vi "Get ColumnName Alais Name.vi"(8 "error in (no error)":errorcluster, 10 "TableName":string="Results", 11 "SQLite in":refnum<class "SQLite.lvclass">) -> (0 "error out":errorcluster, 2 "Columnname_Alais":string[](array[string]), 3 "SQLite out":refnum<class "SQLite.lvclass">)   [LabVIEW 2017, in "SQLite.lvclass"]
uses:
  SQLite.lvclass
  \\vmware-host\Shared Folders/D/Dev/NJAL/OP140/OP140_NJAL_valve_EOL_Test_20210806/Source_Public/DataBase/Top DB/TopDBClass.lvclass
  <userlib>/LabSQL/LabSQL.lvlib
  <userlib>/sushu/sushu.lvlib
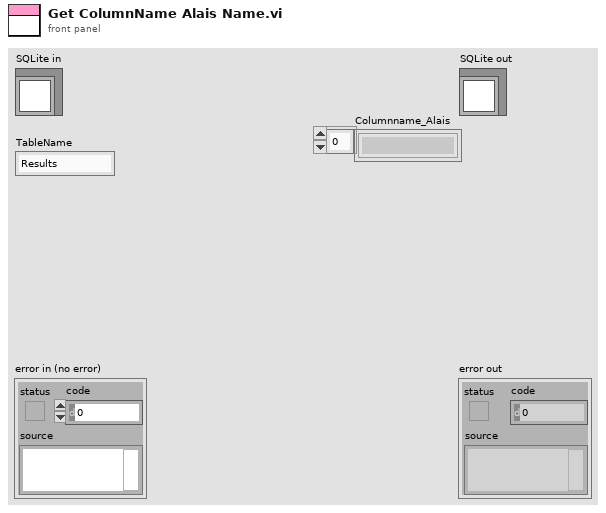
[diagram p1: front panel]
types:
  T1 = enum16{"Other", "SQL2008", "SQLite", "Access", "MySQL"}
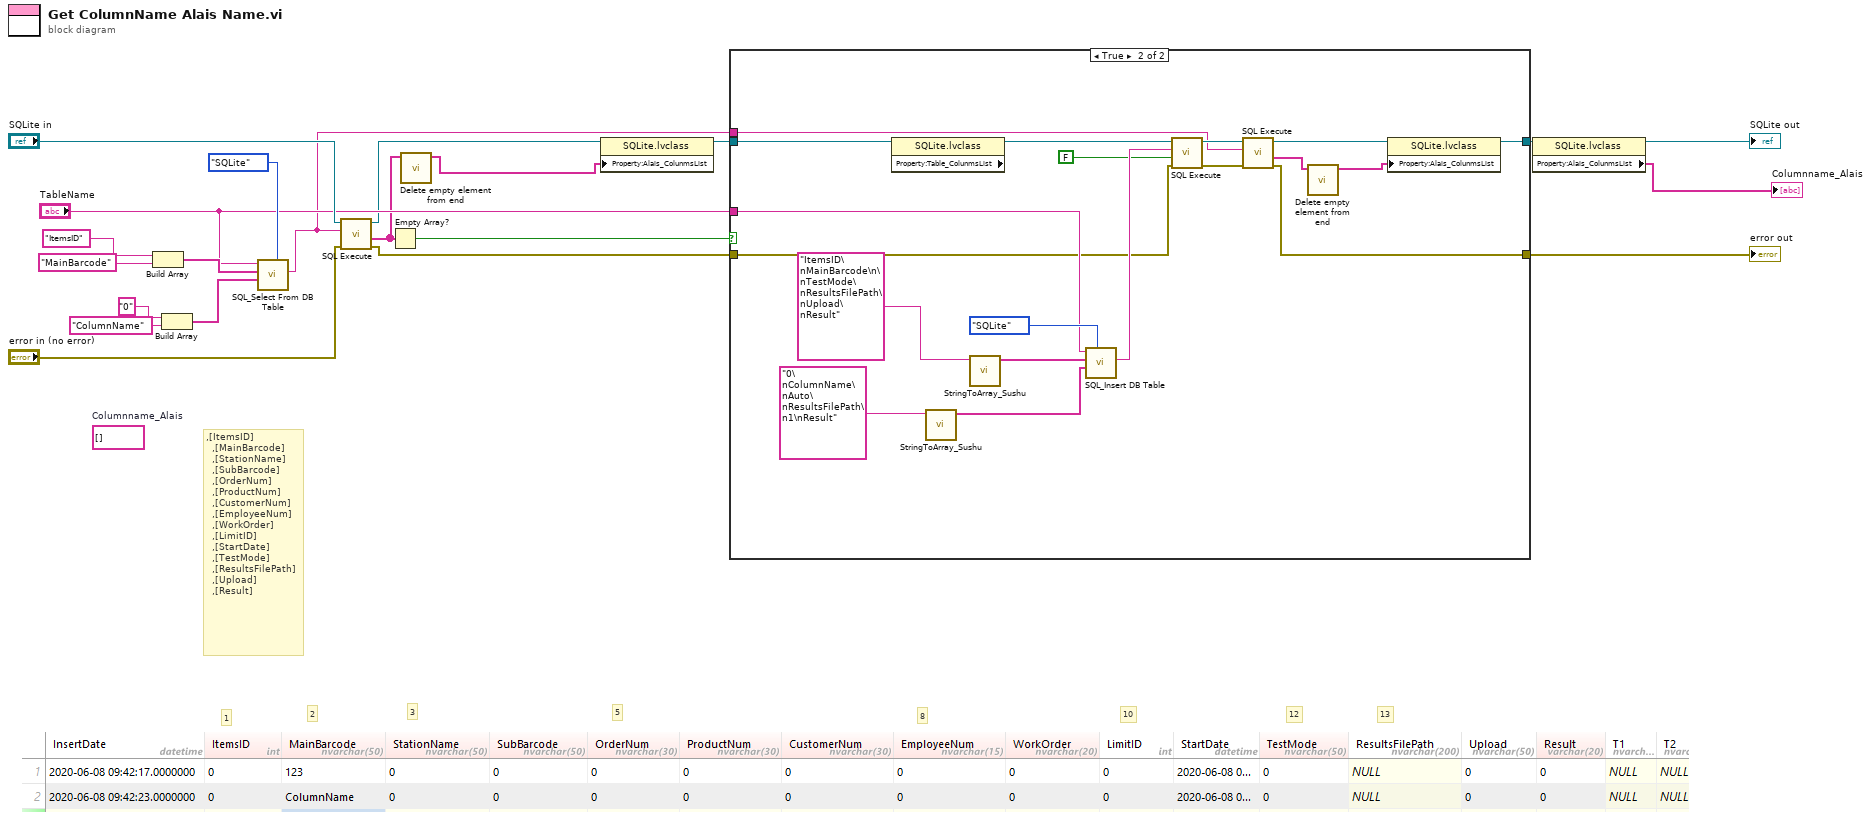
[diagram p0: block diagram]
diagram:
  (unwired) string[] []  # Columnname_Alais
  # "13"
  # "12"
  # "10"
  # "8"
  # "5"
  # "3"
  # "2"
  # "1"
  # ",[ItemsID]\n\t\t,[MainBarcode]\n\t\t,[StationName]\n\t\t,[SubBarcode]\n\t\t,[OrderNum]\n\t\t,[ProductNum]\n\t\t,[CustomerNum]\n\t\t,[EmployeeNum]\n\t\t,[WorkOrder]\n\t\t,[LimitID]\n\t\t,[StartDate]\n\t\t,[TestMode]\n\t\t,[ResultsFilePath]\n\t\t,[Upload]\n\t\t,[Result]"
  n1 = Build Array("ItemsID" ("element"), "MainBarcode" ("element")) -> (w18:string[])
  n2 = Build Array("0" ("element"), "ColumnName" ("element")) -> (w19:string[])
  n3 = call <userlib>:"SQL_Select From DB Table.vi"("DB Type"=T1."SQLite", "ColumnsValue"=w19, "ColumnsNameList"=w18, "TableName"="TableName") -> ("Select SQL CMD"=w8:string)  [unwired: 7 in]
  n4 = call-dynamic "SQL Execute.vi"("error in (no error)"="error in (no error)", "Command Text"=w8, "HostDB in"="SQLite in") -> ("error out"=w11:errorcluster, "FirstRow"=w6:string[], "HostDB out"=w3:refnum<class "SQLite.lvclass">)  [unwired: 4 in, 2 out]
  n5 = Empty Array?(array=w6) -> (empty?=w12:bool)
  n6 = call "Delete empty element from end.vi"("Columnname_Alais"=w6) -> ("reversed array"=w4:string[])  [unwired: 10 in]
  n7 = property class="SQLite.lvclass"(reference=w3, "Property:Alais_ColunmsList"=w4) -> (reference out=w5:refnum<class "SQLite.lvclass">)  [unwired: 1 in, 1 out]
  n8 = case shown="True" w12 {
    tunnel: w5 -> [w23 w39]
    tunnel: [w23 w25] -> w7
    tunnel: w11 -> [w22 w32]
    tunnel: [w22 w28] -> w10
    tunnel: "TableName" -> [_ w37]
    tunnel: w8 -> [_ w30]
    frame False {
    }
    frame True {
      n9 = property class="SQLite.lvclass" props=["Property:Table_ColunmsList"](reference=w39) -> (reference out=w38:refnum<class "SQLite.lvclass">)  [unwired: 1 in, 2 out]
      n10 = call <userlib>:"StringToArray_Sushu.vi"("State Queue"="0\nColumnName\nAuto\nResultsFilePath\n1\nResult") -> ("Array"=w33:string[])  [unwired: 8 in, 2 out]
      n11 = call <userlib>:"StringToArray_Sushu.vi"("State Queue"="ItemsID\nMainBarcode\n\nTestMode\nResultsFilePath\nUpload\nResult") -> ("Array"=w36:string[])  [unwired: 8 in, 2 out]
      n12 = call <userlib>:"SQL_Insert DB Table.vi"("DB Type"=T1."SQLite", "ColumnsValue"=w33, "ColumnsName"=w36, "Table Name"=w37) -> ("Insert DB String"=w42:string)  [unwired: 7 in]
      n13 = call-dynamic "SQL Execute.vi"("error in (no error)"=w32, "Return Data (T)"=FALSE, "Command Text"=w42, "HostDB in"=w38) -> ("error out"=w29:errorcluster, "HostDB out"=w31:refnum<class "SQLite.lvclass">)  [unwired: 3 in, 3 out]
      n14 = call-dynamic "SQL Execute.vi"("error in (no error)"=w29, "Command Text"=w30, "HostDB in"=w31) -> ("error out"=w28:errorcluster, "FirstRow"=w27:string[], "HostDB out"=w26:refnum<class "SQLite.lvclass">)  [unwired: 4 in, 2 out]
      n15 = call "Delete empty element from end.vi"("Columnname_Alais"=w27) -> ("reversed array"=w24:string[])  [unwired: 10 in]
      n16 = property class="SQLite.lvclass"(reference=w26, "Property:Alais_ColunmsList"=w24) -> (reference out=w25:refnum<class "SQLite.lvclass">)  [unwired: 1 in, 1 out]
    }
  }
  "error out" <- w10
  n17 = property class="SQLite.lvclass"(reference=w7) -> (reference out=→"SQLite out":refnum<class "SQLite.lvclass">, "Property:Alais_ColunmsList"=→"Columnname_Alais":string[])  [unwired: 1 in, 1 out]
